vi "pidMotor.vi"(0 "Encoder":string="My Encoder RefNum", 1 "Multiplier":dbl format="%#_13g", 5 "position PID gains":T1={"proportional gain (Kc)"=1.0, "integral time (Ti, min)"=0.01, "derivative time (Td, min)"=0.0} {"derivative time (Td, min)" format="%.3f"; "integral time (Ti, min)" format="%.3f"; "proportional gain (Kc)" format="%.3f"}, 7 "Joystic  cluster":cluster{"X":dbl, "Y":dbl}, 9 "speed mode PID gains":T1={"proportional gain (Kc)"=1.0, "integral time (Ti, min)"=0.01, "derivative time (Td, min)"=0.0} {"derivative time (Td, min)" format="%.3f"; "integral time (Ti, min)" format="%.3f"; "proportional gain (Kc)" format="%.3f"}, 11 "error in (no error)":errorcluster, 12 "Init?":bool) -> (4 "output":dbl, 6 "minimum % vbus":dbl, 10 "Rate":dbl, 14 "Distance":dbl, 15 "error out":errorcluster)   [LabVIEW 2013]
uses:
  <vilib>/addons/control/pid/pid.llb/PID (DBL).vi
  <vilib>/addons/control/pid/pid.llb/PID Control Input Filter (DBL).vi
  <vilib>/addons/control/pid/NI_PID_pid.lvlib
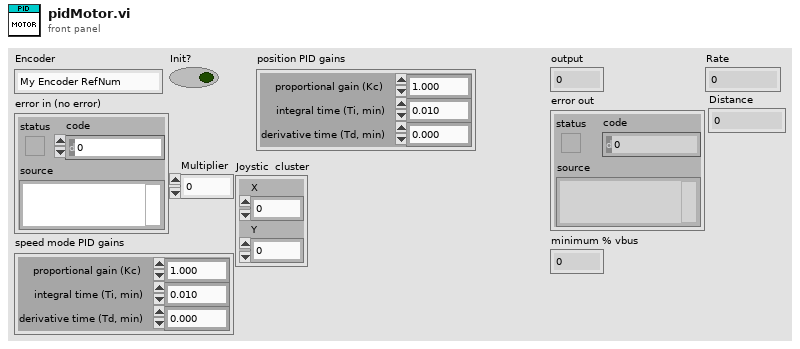
[diagram p1: front panel]
types:
  T1 = cluster{"proportional gain (Kc)":dbl, "integral time (Ti, min)":dbl, "derivative time (Td, min)":dbl}
  T2 = typedef "WPI_EncoderDevRef.ctl" = cluster{"DevStatus":errorcluster, "EncoderIndex":T3, "CounterIndex":T4, "DistancePerCount":dbl, "Decoding Type":T5}
  T3 = typedef "FPGA_EncoderIdx.ctl" = enum8{"Enc 0", "Enc 1", "Enc 2", "Enc 3", "Invalid"}
  T4 = typedef "FPGA_CounterCtrSystemIndex.ctl" = enum8{"Ctr 0", "Ctr 1", "Ctr 2", "Ctr 3", "Ctr 4", "Ctr 5", "Ctr 6", "Ctr 7", "Invalid"}
  T5 = typedef "WPI_EncoderType.ctl" = enum16{"1x", "2x", "4x"}
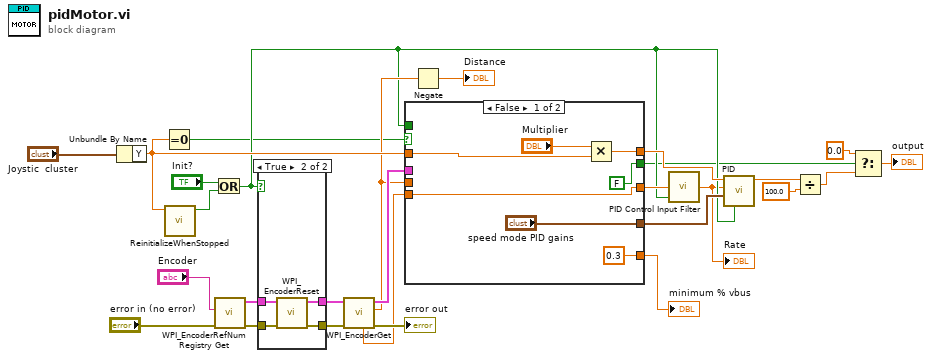
[diagram p0: block diagram]
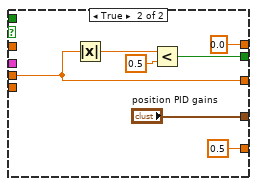
[diagram p3: hidden frame]
diagram:
  n1 = Unbundle By Name("Joystic  cluster") -> ("Y"=w25:dbl)
  n2 = Equal To 0?(x=w25) -> (x = 0?=w2:bool)
  n3 = call "ReinitializeWhenStopped.vi"("JoystickValue"=w25) -> ("reinitialize? (F)"=w11:bool)  [unwired: 10 in]
  n4 = Or(x="Init?", y=w11) -> (x .or. y?=w10:bool)
  n5 = call <vilib>:"WPI_EncoderRefNum Registry Get.vi"("error in (no error)"="error in (no error)", "refnum name"="Encoder") -> ("error out"=w21:errorcluster, "EncoderDevRef"=w22:T2)  [unwired: 8 in]
  n6 = case shown="True" w10 {
    tunnel: w21 -> [w29 w34]
    tunnel: w22 -> [w30 w33]
    tunnel: [w30 w32] -> w20
    tunnel: [w29 w31] -> w19
    frame False {
    }
    frame True {
      n7 = call <vilib>:"WPI_EncoderReset.vi"("error in (no error)"=w34, "EncoderDevRef"=w33) -> ("error out"=w31:errorcluster, "EncoderDevRef"=w32:T2)  [unwired: 8 in]
    }
  }
  n8 = call <vilib>:"WPI_EncoderGet.vi"("error in (no error)"=w19, "EncoderDevRef"=w20) -> ("error out"=→"error out":errorcluster, "Distance"=w14:dbl, "EncoderDevRef"=w24:T2, "Rate"=w13:dbl)  [unwired: 4 in, 2 out]
  n9 = case shown="False" w2 {
    tunnel: w13 -> [w37 _]
    tunnel: w25 -> [w40 _]
    tunnel: w10 -> [_ _]
    tunnel: w24 -> [_ _]
    tunnel: w14 -> [_ w47]
    tunnel: ["speed mode PID gains" "position PID gains"] -> w16
    tunnel: [w38 0.0] -> w15
    tunnel: [w37 w47] -> w12
    tunnel: [FALSE w43] -> w4
    tunnel: [0.3 ("f") 0.5 ("t")] -> w1
    frame False {
      n10 = Multiply(x="Multiplier", y=w40) -> (x*y=w38:dbl)
    }
    frame True {
      n11 = Absolute Value(x=w47) -> (abs(x)=w46:dbl)
      n12 = Less?(x=w46, y=0.5) -> (x < y?=w43:bool)
    }
  }
  "minimum % vbus" <- w1
  n13 = Negate(x=w14) -> (-x=→"Distance":dbl)
  n14 = call-poly <vilib>:"PID Control Input Filter.vi"("reinitialize? (F)"=w10, "input"=w12) -> ("output"=w3:dbl)  [unwired: 3 in]
  "Rate" <- w3
  n15 = call-poly <vilib>:"PID.vi"("reinitialize? (F)"=w10, "PID gains"=w16, "process variable"=w3, "setpoint"=w15) -> ("output"=w17:dbl)  [unwired: 6 in, 1 out]
  n16 = Divide(x=w17, y=100.0) -> (x/y=w6:dbl)
  n17 = Select(t=0.0 ("output"), s=w4, f=w6) -> (s? t:f=→"output":dbl)
